vi "SubVI Is Password Locked.vi"(8 "Error In":errorcluster, 11 "SubVI ref":refnum<vi>) -> (0 "Error Out":errorcluster, 3 "isPasswordLocked?":bool)   [LabVIEW 2014]
doc: "Return TRUE if SubVI is locked by password. Otherwise FALSE."
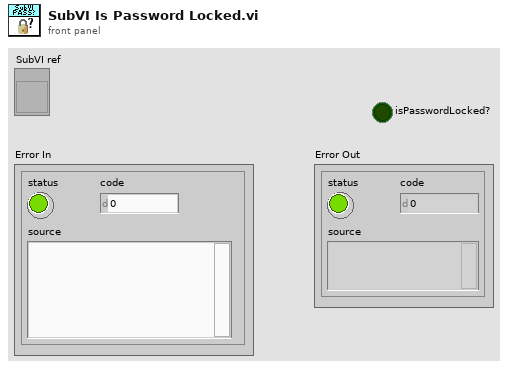
[diagram p1: front panel]
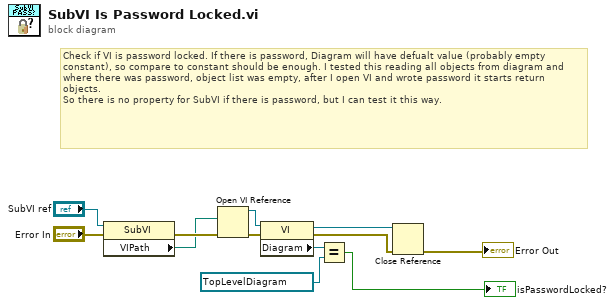
[diagram p0: block diagram]
diagram:
  # "Check if VI is password locked. If there is password, Diagram will have defualt value (probably empty constant), so compare to constant should be enough. I tested this reading all objects from diagram and where there was password, object list was empty, after I open VI and wrote password it starts return objects.\nSo there is no property for SubVI if there is password, but I can test it this way."
  n1 = property class="SubVI"(reference="SubVI ref", error in="Error In") -> (error out=w3:errorcluster, "VIPath"=w2:path)  [unwired: 1 out]
  n2 = Open VI Reference(vi path=w2, error in (no error)=w3) -> (vi reference=w11:refnum<vi>, error out=w12:errorcluster)  [unwired: 4 in]
  n3 = property on="Property Node" class="VI"(reference=w11, error in=w12) -> (reference out=w6:refnum<vi>, error out=w7:errorcluster, "Diagram"=w9:refnum<vi>)
  n4 = Equal?(x=w9, y=refnum<vi> refnum ("Block Diagram")) -> (x = y?=→"isPasswordLocked?":bool)
  n5 = Close Reference(reference=w6, error in (no error)=w7) -> (error out=→"Error Out":errorcluster)
